vi "motorPosControl (SubVI).vi"(6 "Reset":bool, 7 "+/- Range":dbl, 8 "error in (no error)":errorcluster, 9 "PID gains":T1={"proportional gain (Kc)"=2.0, "integral time (Ti, min)"=0.01, "derivative time (Td, min)"=0.00010000000000000003}, 10 "Position (deg)":dbl, 11 "dt":i64) -> (0 "error out":errorcluster, 1 "Waveform Chart":T2(graph), 2 "MotorEncoder (deg)":dbl, 4 "out of range!":bool)   [LabVIEW 2019, in "SJCube_KNRm.lvlib"]
uses:
  SJCube_KNRm.lvlib
  <vilib>/addons/control/pid/pid.llb/PID (DBL).vi
  <vilib>/addons/control/pid/NI_PID_pid.lvlib
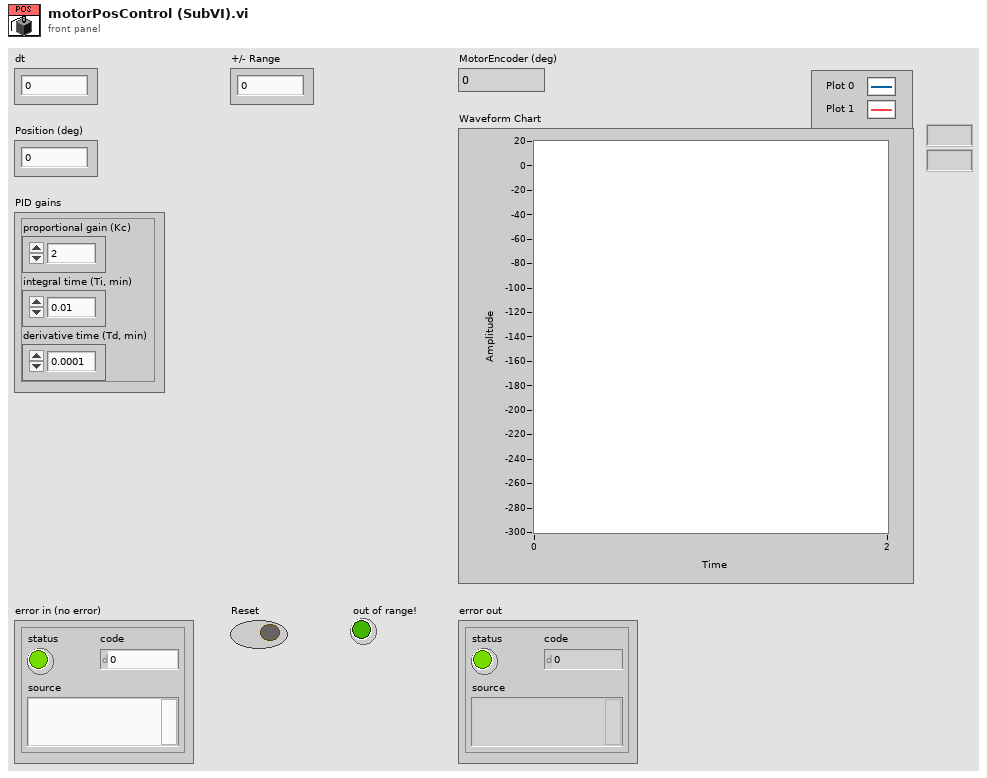
[diagram p1: front panel]
types:
  T1 = cluster{"proportional gain (Kc)":dbl, "integral time (Ti, min)":dbl, "derivative time (Td, min)":dbl}
  T2 = cluster{"Position (deg)":dbl, "MotorEncoder (deg)":dbl}
  T3 = cluster{"+/- Range":dbl, "MotorEncoder (deg)":dbl}
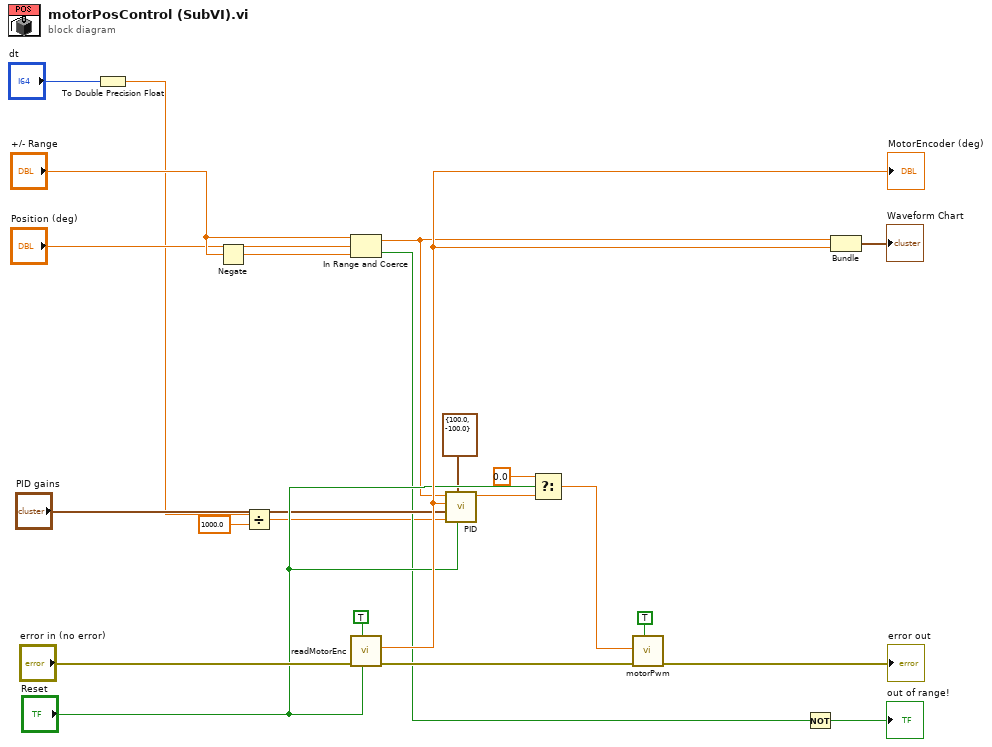
[diagram p0: block diagram]
diagram:
  n1 = To Double Precision Float(number="dt") -> (double precision float=w3:dbl)
  n2 = Negate(x="+/- Range") -> (-x=w10:dbl)
  n3 = Divide(x=w3, y=1000.0) -> (x/y=w1:dbl)
  n4 = In Range and Coerce(upper limit="+/- Range", x="Position (deg)", lower limit=w10) -> (coerced(x)=w7:dbl, In Range?=w6:bool)
  n5 = call "readMotorEnc.vi"("Reset Counter"="Reset", "Reverse ENC?"=TRUE, "error in (no error)"="error in (no error)") -> ("error out"=w15:errorcluster, "MotorEncoder (deg)"=w21:dbl)  [unwired: 7 in]
  "MotorEncoder (deg)" <- w21
  n6 = call-poly <vilib>:"PID.vi"("reinitialize? (F)"="Reset", "output range"=cluster{"output high":dbl, "output low":dbl} {"output high"=100.0, "output low"=-100.0}, "dt (s)"=w1, "PID gains"="PID gains", "process variable"=w21, "setpoint"=w7) -> ("output"=w19:dbl)  [unwired: 4 in, 1 out]
  n7 = Select(t=0.0, s="Reset", f=w19) -> (s? t:f=w20:dbl)
  n8 = call "motorPwm.vi"("reverse?"=TRUE, "error in (no error)"=w15, "Speed (PWM)"=w20) -> ("error out"=→"error out":errorcluster)  [unwired: 8 in]
  n9 = Not(x=w6) -> (.not. x?=→"out of range!":bool)
  n10 = Bundle("+/- Range"=w7, "MotorEncoder (deg)"=w21) -> (→"Waveform Chart":T3)  [unwired: 1 in]
